vi "Verify DTC.vi"(6 "Expected DTC":string, 8 "error in":errorcluster, 9 "Address":string, 10 "Address Lookup Table":variant, 11 "connection info":T2) -> (0 "error out":errorcluster, 1 "Status":T4, 2 "Address Lookup Table Out":variant, 3 "connection info":T2, 4 "Found DTCs":i32)   [LabVIEW 2019, in "J1939 Host Automation API.lvlib"]
uses:
  J1939 Host Automation API.lvlib
  <vilib>/NI/STM/TCP/TCP Connection Info.ctl
  <vilib>/NI/STM/SubVIs/MetaDataElement.ctl
  Addon/Addon Shared/Types/Verify DTC_Status.ctl
  Addon/Addon Shared/Types/Convert DTCs Cluster.ctl
  Addon/Addon Shared/J1939 Addon Shared.lvlib
  <vilib>/NI/STM/NI STM.lvlib
panel:
  out "Responses":T1[](array[typedef])
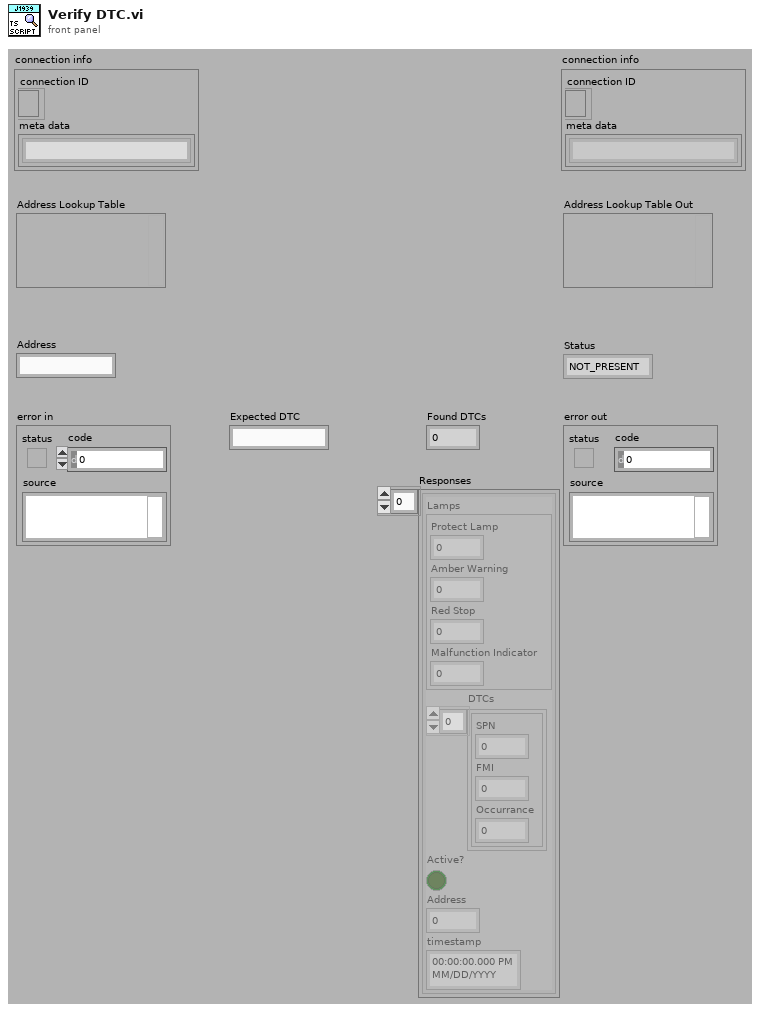
[diagram p1: front panel]
types:
  T1 = typedef "J1939 Addon Shared.lvlib/Convert DTCs Cluster.ctl" = cluster{"Lamps":cluster{"Protect Lamp":u8, "Amber Warning":u8, "Red Stop":u8, "Malfunction Indicator":u8}, "DTCs":cluster{"SPN":u32, "FMI":u8, "Occurrance":u8}[], "Active?":bool, "Address":u8, "timestamp":timestamp}
  T2 = typedef "NI STM.lvlib/TCP Connection Info.ctl" = cluster{"connection ID":refnum<k5>, "meta data":T3[]}
  T3 = typedef "NI STM.lvlib/MetaDataElement.ctl" = string
  T4 = typedef "J1939 Addon Shared.lvlib/Verify DTC_Status.ctl" = enum16{"NOT_PRESENT", "ACTIVE", "INACTIVE"}
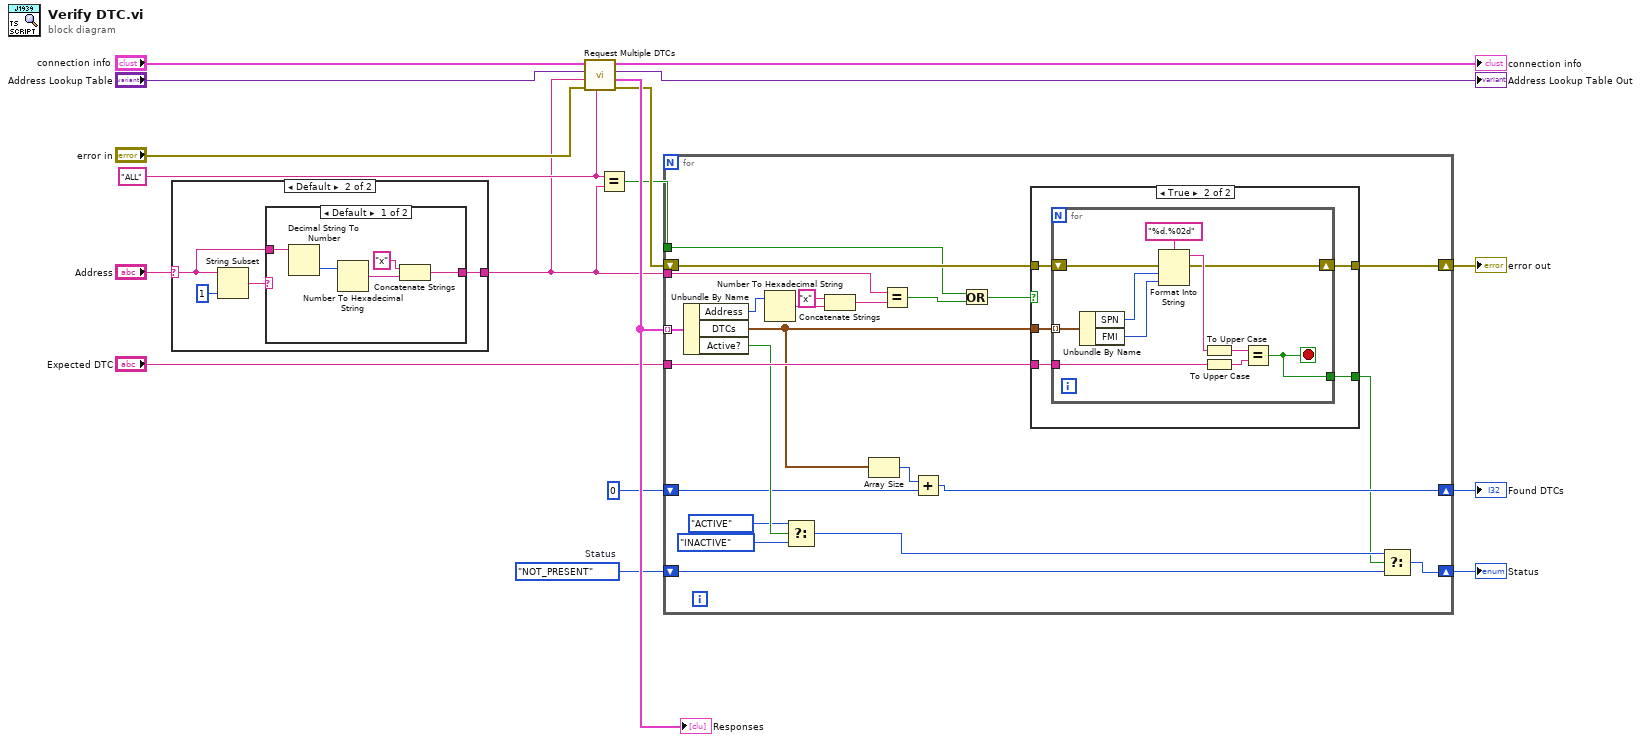
[diagram p0: block diagram]
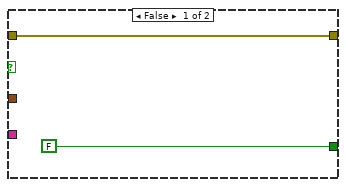
[diagram p4: hidden frame]
diagram:
  w4 = "ALL" ("TLA (ALL)")
  w11 = Verify_DTC_Status."NOT_PRESENT"  # Status
  n1 = case shown="Default" "Address" {
    selector: "Address" -> [w18 w20]
    tunnel: [w18 w19] -> w1
    frame "ALL" {
    }
    frame Default {
      n2 = String Subset(string=w20, length (rest)=1 ("length (rest)")) -> (substring=w21:string)  [unwired: 1 in]
      n3 = case shown="Default" w21 {
        tunnel: w20 -> [w27 w28]
        tunnel: [w23 w28] -> w19
        frame Default {
          n4 = Decimal String To Number(string=w27) -> (number=w26:i32)  [unwired: 2 in, 1 out]
          n5 = Number To Hexadecimal String(2:w26) -> (0:w25:string)  [unwired: 1 in]
          n6 = Concatenate Strings("x" ("string"), w25) -> (w23:string)
        }
        frame "x" {
        }
      }
    }
  }
  n7 = call "Request Multiple DTCs.vi"("Command"=w4, "error in"="error in", "Address"=w1, "Lookup Table"="Address Lookup Table", "connection info"="connection info") -> ("error out"=w9:errorcluster, "Responses"=w13:T1[], "Lookup Table Out"=→"Address Lookup Table Out":variant, "connection info"=→"connection info":T2)  [unwired: 2 in, 1 out]
  "Responses" <- w13
  n8 = Equal?(x=w4, y=w1) -> (x = y?=w3:bool)
  n9 = for {
    tunnel: w13 -> [w51] mode=indexing
    tunnel: "Expected DTC" -> [w50]
    shift-right: [w44] -> w10
    shift-left: w11 -> [w45]
    shift-right: [w42] -> w8
    shift-left: w9 -> [w43]
    tunnel: w1 -> [w41]
    shift-right: [w35] -> w5
    shift-left: 0 -> [w37]
    tunnel: w3 -> [w31]
    n10 = Unbundle By Name(w51) -> ("Address"=w39:u8, "DTCs"=w38:cluster{"SPN":u32, "FMI":u8, "Occurrance":u8}[], "Active?"=w49:bool)
    n11 = Number To Hexadecimal String(2:w39) -> (0:w40:string)  [unwired: 1 in]
    n12 = Select(t=Verify_DTC_Status."ACTIVE" ("Status"), s=w49, f=Verify_DTC_Status."INACTIVE" ("Status")) -> (s? t:f=w46:T4)
    n13 = Concatenate Strings("x" ("string"), w40) -> (w30:string)
    n14 = Array Size(array=w38) -> (size(s)=w36:i32)
    n15 = Equal?(x=w41, y=w30) -> (x = y?=w34:bool)
    n16 = Add(x=w36, y=w37) -> (x+y=w35:i32)
    n17 = Or(x=w31, y=w34) -> (x .or. y?=w32:bool)
    n18 = case shown="True" w32 {
      tunnel: w38 -> [_ w58]
      tunnel: w50 -> [_ w57]
      tunnel: [FALSE w56] -> w33
      tunnel: w43 -> [w53 w55]
      tunnel: [w53 w54] -> w42
      frame False {
      }
      frame True {
        n19 = for {
          tunnel: w58 -> [w66] mode=indexing
          tunnel: w57 -> [w64]
          tunnel: [w61] -> w56
          shift-right: [w59] -> w54
          shift-left: w55 -> [w60]
          stop <- w61 stop-if-true
          n20 = Unbundle By Name(w66) -> ("SPN"=w69:u32, "FMI"=w68:u8)
          n21 = Format Into String(format string="%d.%02d", error in=w60, w69, w68) -> (resulting string=w65:string, error out=w59:errorcluster)  [unwired: 1 in]
          n22 = To Upper Case(1:w65) -> (0:w63:string)
          n23 = To Upper Case(1:w64) -> (0:w62:string)
          n24 = Equal?(x=w63, y=w62) -> (x = y?=w61:bool)
        }
      }
    }
    n25 = Select(t=w46, s=w33, f=w45) -> (s? t:f=w44:T4)
  }
  "Status" <- w10
  "Found DTCs" <- w5
  "error out" <- w8
